vi "Drive_Sensor_To_Angle.vi"(1 "Position (Raw Sensor Units)":i32) -> (0 "Numeric":dbl)   [LabVIEW 2019]
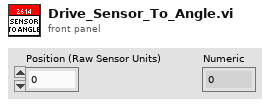
[diagram p1: front panel]
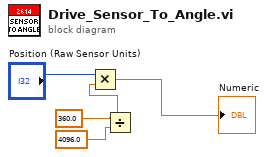
[diagram p0: block diagram]
diagram:
  n1 = Divide(x=360.0, y=4096.0) -> (x/y=w4:dbl)
  n2 = Multiply(x="Position (Raw Sensor Units)", y=w4) -> (x*y=→"Numeric":dbl)
